vi "SaveVi.vi"(8 "error in":errorcluster, 11 "State":T1) -> (0 "error out":errorcluster, 3 "State out":T1)   [LabVIEW 2013, in "control module data interface generator.lvlib"]
uses:
  control module data interface generator.lvlib
  Controls/StateCluster.ctl
  Controls/initialized references.ctl
  Controls/interface VI type.ctl
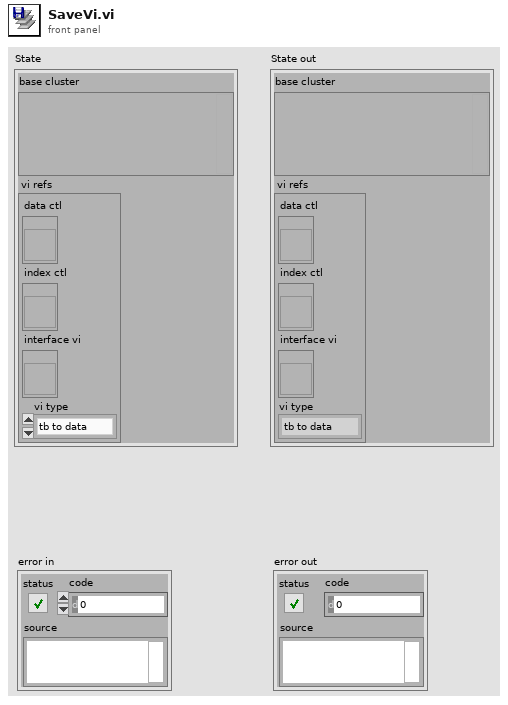
[diagram p1: front panel]
types:
  T1 = typedef "control module data interface generator.lvlib/StateCluster.ctl" = cluster{"base cluster":variant, "vi refs":T2}
  T2 = typedef "control module data interface generator.lvlib/initialized references.ctl" = cluster{"data ctl":refnum<vi>, "index ctl":refnum<vi>, "interface vi":refnum<vi>, "vi type":T3}
  T3 = typedef "control module data interface generator.lvlib/interface VI type.ctl" = enum16{"tb to data", "data to tb"}
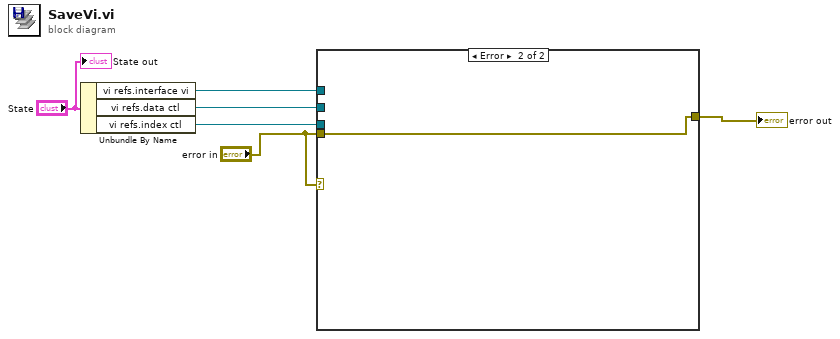
[diagram p0: block diagram]
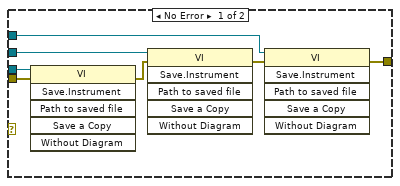
[diagram p2: hidden frame]
diagram:
  n1 = Unbundle By Name("State") -> ("vi refs.interface vi"=w6:refnum<vi>, "vi refs.data ctl"=w3:refnum<vi>, "vi refs.index ctl"=w2:refnum<vi>)
  n2 = case shown="Error" "error in" {
    tunnel: w6 -> [w13 _]
    tunnel: [w12 w14] -> w4
    tunnel: w3 -> [w11 _]
    tunnel: w2 -> [w10 _]
    tunnel: "error in" -> [w9 w14]
    frame No Error {
      n3 = invoke class="VI" method="Save.Instrument"(reference=w10, error in=w9) -> (error out=w8:errorcluster)  [unwired: 4 in, 5 out]
      n4 = invoke class="VI" method="Save.Instrument"(reference=w11, error in=w8) -> (error out=w7:errorcluster)  [unwired: 4 in, 5 out]
      n5 = invoke class="VI" method="Save.Instrument"(reference=w13, error in=w7) -> (error out=w12:errorcluster)  [unwired: 4 in, 5 out]
    }
    frame Error {
    }
  }
  "error out" <- w4
  "State out" <- "State"
